vi "Check for Message.vi"(8 "error in":errorcluster) -> (0 "error out":errorcluster)   [LabVIEW 2015]
uses:
  Modules/myPAM/Private TypeDefs/Module Reference.ctl
  Global TypeDefs/Registered Modules.ctl
  Modules/myPAM/Private TypeDefs/Module Queues.ctl
  Modules/myPAM/Private TypeDefs/Message Queue Element.ctl
  Modules/myPAM/Public TypeDefs/Messages.ctl
  Modules/myPAM/Private TypeDefs/Module Notifiers.ctl
  Modules/myPAM/Private TypeDefs/Dummy Notifier.ctl
  Modules/myPAM/myPAM.lvlib
panel:
  out "new element available":bool
  in  "module reference":T1
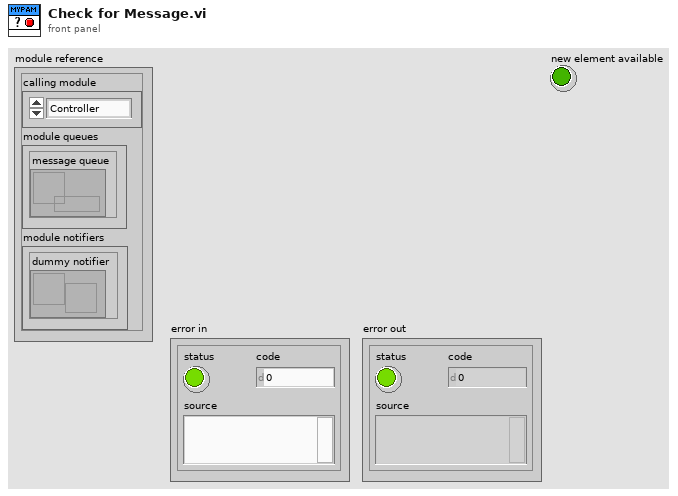
[diagram p1: front panel]
types:
  T1 = typedef "myPAM.lvlib/Module Reference.ctl" = cluster{"calling module":T2, "module queues":T3, "module notifiers":T4}
  T2 = typedef "Registered Modules.ctl" = enum16{"Controller", "DAQ", "Error Handler", "Game", "myPAM", "WinHost", "Logger"}
  T3 = typedef "myPAM.lvlib/Module Queues.ctl" = cluster{"message queue":refnum<queue>}
  T4 = typedef "myPAM.lvlib/Module Notifiers.ctl" = cluster{"dummy notifier":refnum<notifier>}
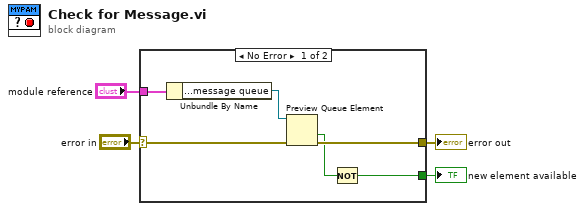
[diagram p0: block diagram]
diagram:
  n1 = case shown="No Error" "error in" {
    selector: "error in" -> [w10 w11]
    tunnel: "module reference" -> [w9 _]
    tunnel: [w7 w11] -> w2
    tunnel: [w5 _] -> w1
    frame No Error {
      n2 = Unbundle By Name(w9) -> ("module queues.message queue"=w8:refnum<queue>)
      n3 = Preview Queue Element(queue=w8, error in (no error)=w10) -> (timed out?=w6:bool, error out=w7:errorcluster)  [unwired: 1 in, 2 out]
      n4 = Not(x=w6) -> (.not. x?=w5:bool)
    }
    frame Error {
    }
  }
  "error out" <- w2
  "new element available" <- w1
